vi "Set Parameters.vi"(8 "error in (no error)":errorcluster, 10 "Parameters":T1, 11 "Execution in":refnum<class "Execution.lvclass">) -> (0 "error out":errorcluster, 3 "Execution out":refnum<class "Execution.lvclass">)   [LabVIEW 2020, in "TSS.lvlib" / "Execution.lvclass"]
uses:
  Execution.lvclass
  VariableContainer/Typedefs/Session Handle.ctl
  VariableContainer/VariableContainer.lvclass
  Execution.lvclass/Execution.ctl
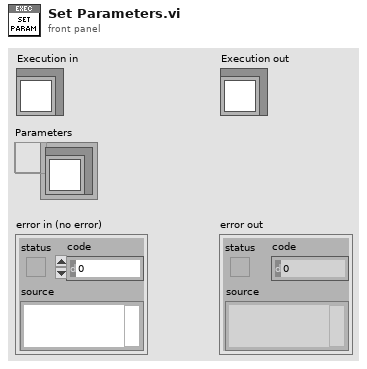
[diagram p1: front panel]
types:
  T1 = typedef "TSS.lvlib/VariableContainer.lvclass/Session Handle.ctl" = refnum<data-value>
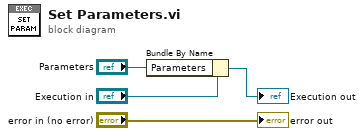
[diagram p0: block diagram]
diagram:
  n1 = Bundle By Name(cluster="Execution in", "Parameters"="Parameters") -> (→"Execution out":refnum<class "Execution.lvclass">)
  "error out" <- "error in (no error)"
